vi "VerifyAnswer.vi"(1 "answer":dbl, 2 "guess":dbl, 3 "tolerance(%)":dbl) -> (0 "correct?":bool)   [LabVIEW 2014]
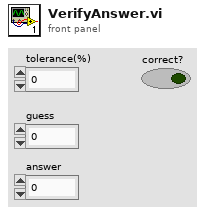
[diagram p1: front panel]
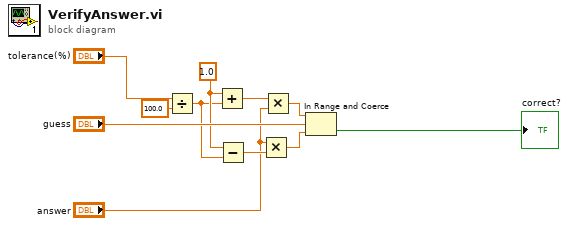
[diagram p0: block diagram]
diagram:
  w2 = 1.0 ("y")
  n1 = Divide(x="tolerance(%)", y=100.0) -> (x/y=w1:dbl)
  n2 = Add(x=w2, y=w1) -> (x+y=w7:dbl)
  n3 = Subtract(x=w2, y=w1) -> (x-y=w8:dbl)
  n4 = Multiply(x="answer", y=w8) -> (x*y=w10:dbl)
  n5 = Multiply(x=w7, y="answer") -> (x*y=w11:dbl)
  n6 = In Range and Coerce(upper limit=w11, x="guess", lower limit=w10) -> (In Range?=→"correct?":bool)  [unwired: 1 out]
